vi "sendStop.vi"(8 "error in (no error)":errorcluster, 11 "WinX32Camera in":refnum<class "WinX32Camera.lvclass">) -> (0 "error out":errorcluster, 3 "WinX32Camera out":refnum<class "WinX32Camera.lvclass">)   [LabVIEW 2011, in "WinX32Camera.lvclass"]
uses:
  WinX32Camera.lvclass
  WinX32Camera.lvclass/WinX32Camera.ctl
  Tools/Filing/FileSystem/FileSystem.lvclass
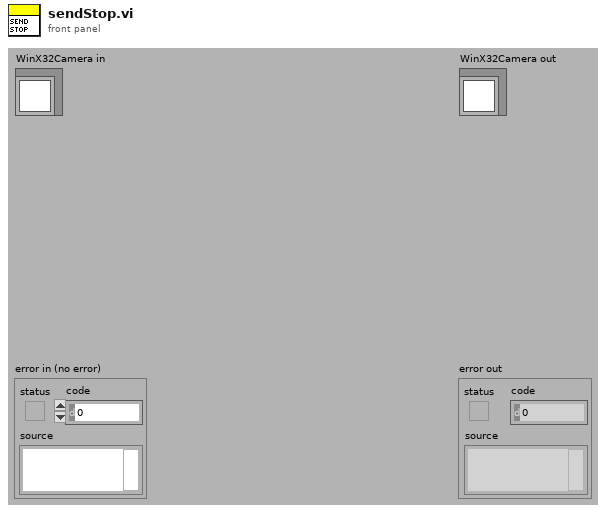
[diagram p1: front panel]
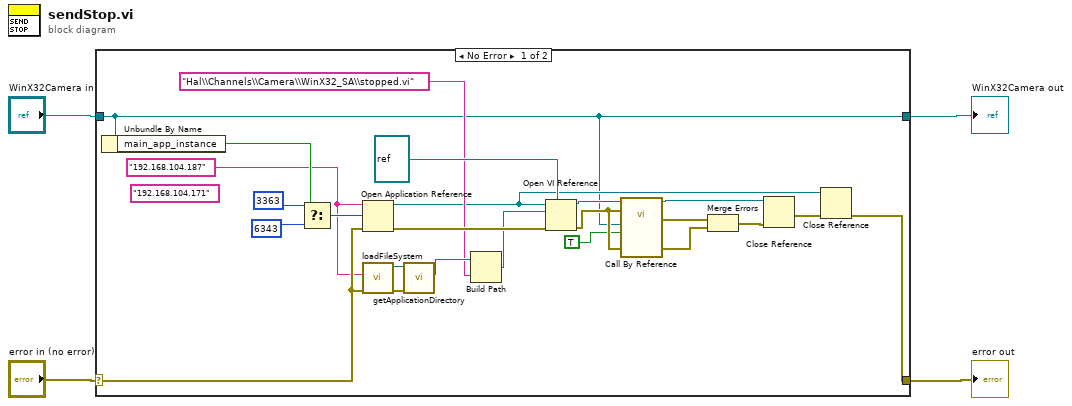
[diagram p0: block diagram]
diagram:
  n1 = case shown="No Error" "error in (no error)" {
    selector: "error in (no error)" -> [w25 w30]
    tunnel: [w13 w30] -> w1
    tunnel: [w11 w29] -> w2
    tunnel: "WinX32Camera in" -> [w11 w29]
    frame No Error {
      (unwired) "192.168.104.171" ("machine name (\"\":  open local reference)")
      w5 = "192.168.104.187" ("machine name (\"\":  open local reference)")
      n2 = Unbundle By Name(w11) -> ("main_app_instance"=w10:bool)
      n3 = Select(t=u16 3363 ("port number or service name (3363)"), s=w10, f=u16 6343 ("port number or service name (3363)")) -> (s? t:f=w7:u16)
      n4 = Open Application Reference(8:w25, 10:w7, 11:w5) -> (0:w28:errorcluster, 3:w15:refnum<vi>)  [unwired: 1 in]
      n5 = call "loadFileSystem.vi"("error in (no error)"=w25, "computer name"=w5) -> ("error out"=w26:errorcluster, "FileSystem out"=w12:refnum<class "FileSystem.lvclass">)  [unwired: 8 in]
      n6 = call-dynamic "getApplicationDirectory.vi"("error in (no error)"=w26, "FileSystem.lvclass in"=w12) -> ("ApplicationDirectory"=w24:path)  [unwired: 7 in, 2 out]
      n7 = Build Path(base path=w24, name or relative path="Hal\\Channels\\Camera\\WinX32_SA\\stopped.vi" ("viPath")) -> (appended path=w22:path)
      n8 = Open VI Reference(type specifier VI Refnum (for type only)=refnum<vi> refnum, application reference (local)=w15, vi path=w22, error in (no error)=w28) -> (vi reference=w21:refnum<vi>, error out=w20:errorcluster)  [unwired: 2 in]
      n9 = call-by-ref "?"(reference=w21, error in=w20, 8:"error in (no error)"=w20, "stopped"=TRUE, "WinX32Camera in"=w11) -> (reference out=w17:refnum<vi>, error out=w19:errorcluster, 0:"error out"=w18:errorcluster)  [unwired: 7 in, 1 out]
      n10 = Merge Errors(w19, w18) -> (w16:errorcluster)
      n11 = Close Reference(reference=w17, error in (no error)=w16) -> (error out=w14:errorcluster)
      n12 = Close Reference(reference=w15, error in (no error)=w14) -> (error out=w13:errorcluster)
    }
    frame Error {
    }
  }
  "error out" <- w1
  "WinX32Camera out" <- w2
